vi "CoffeeMachine.vi"() -> ()   [LabVIEW 2020]
uses:
  Coffee Machine/ClusterConst.ctl
  Coffee Machine/Typedef/QueueOperations.ctl
  <vilib>/Utility/config.llb/Read Key (Double).vi
  <vilib>/Utility/config.llb/Read Key (I32).vi
  <vilib>/Utility/config.llb/Read Key (Boolean).vi
  <vilib>/Utility/config.llb/NI_LVConfig.lvlib
panel:
  out "error out":errorcluster
  in  "error in":errorcluster
  in  "Power":bool
  out "Total Cups":i32
  out "Elapsed Time":dbl
  out "Dispensing":bool
  out "Brewing":bool
  out "Grinding":bool
  out "Heating":bool
  out "Purging":bool
  out "Dispenser":dbl(slide) scale=0.0..10.0
  out "Chamber":dbl(slide) scale=0.0..10.0
  out "Low Milk":bool
  out "Low Bean":bool
  out "Low Water":bool
  out "Milk Level":dbl(slide) scale=0.0..100.0
  out "Bean Level":dbl(slide) scale=0.0..100.0
  out "Water Level":dbl(slide) scale=0.0..100.0
  in  "Type":i32(knob) scale=0.0..2.0
  in  "1-Carafe":bool
  in  "1- Cup":bool
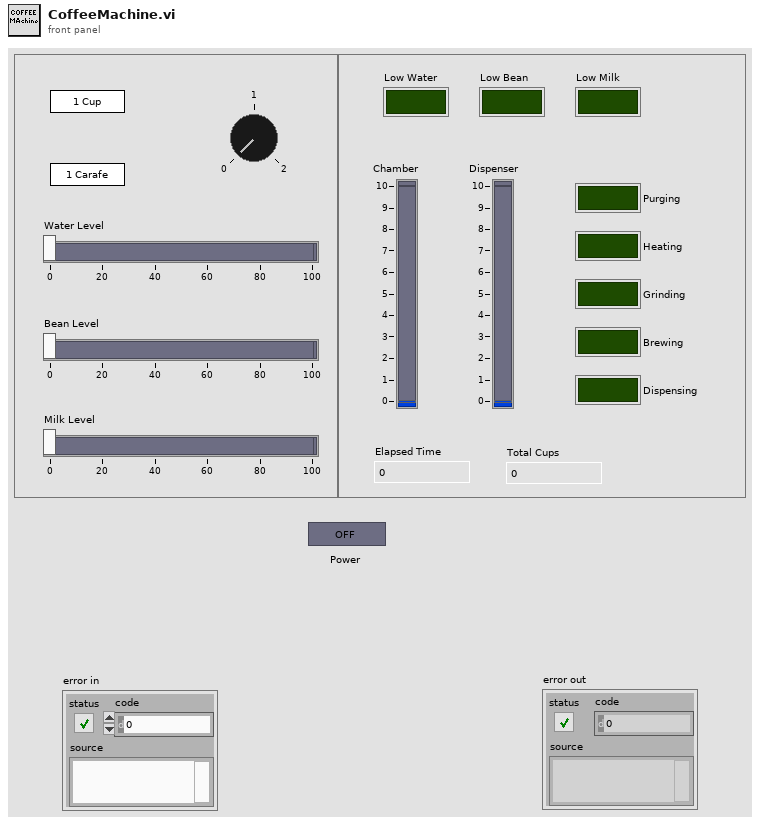
[diagram p1: front panel]
types:
  T1 = typedef "QueueOperations.ctl" = enum16{"Create", "Enqueue", "Enqueue N elements", "Dequeue", "Flush", "Release"}
  T2 = typedef "ClusterConst.ctl" = cluster{"1- Cup":bool, "1-Carafe":bool, "Water Level":dbl, "Bean Level":dbl, "Milk Level":dbl, "Purging":bool, "Heating":bool, "Grinding":bool, "Brewing":bool, "Dispensing":bool, "Chamber ":dbl, "Dispenser":dbl, "Low Water":bool, "Low Bean":bool, "Low Milk":bool, "Elapsed Time":dbl, "Total Cups":i32, "Power":bool, "Type":i32, "Level Array":dbl[], "Shutdown Status":bool, "Time Elapse":dbl, "Start Time":dbl, "Start 1 Seq":i32[], "Start 2 Seq":i32[], "Index":i32}
  T3 = typedef "NI_LVConfig.lvlib/Config Data RefNum.ctl" = refnum<k1>
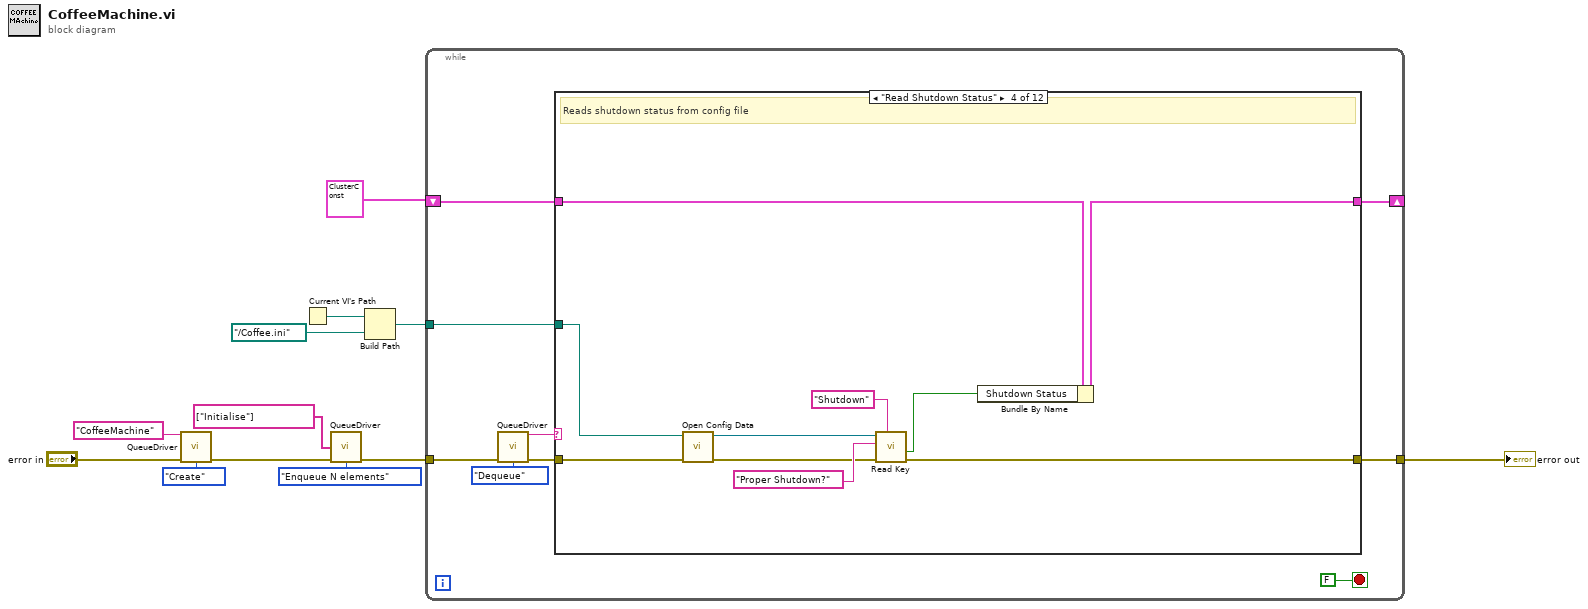
[diagram p0: block diagram]
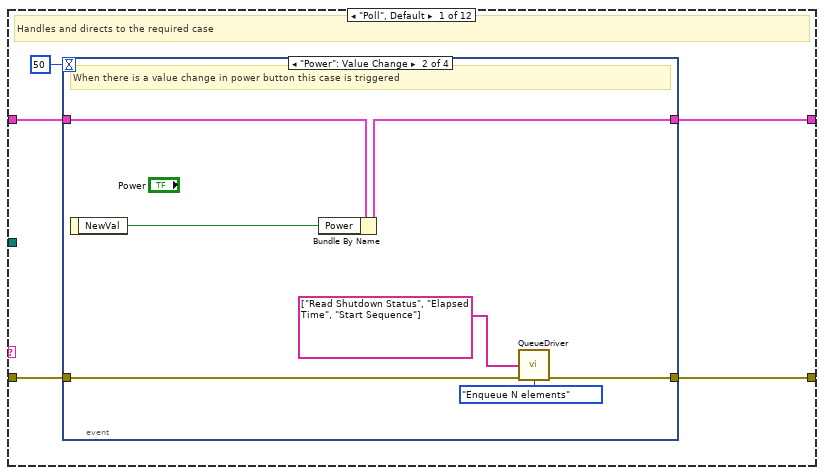
[diagram p2: hidden frame]
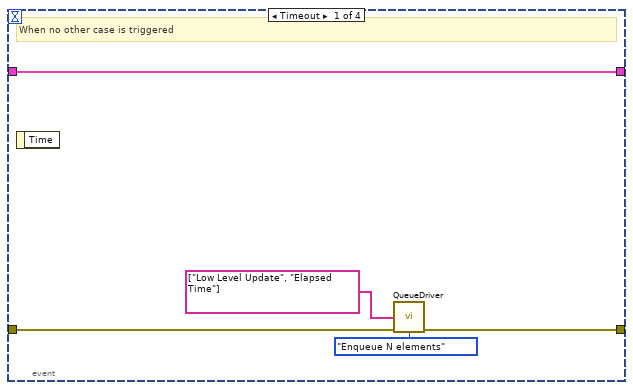
[diagram p3: hidden frame]
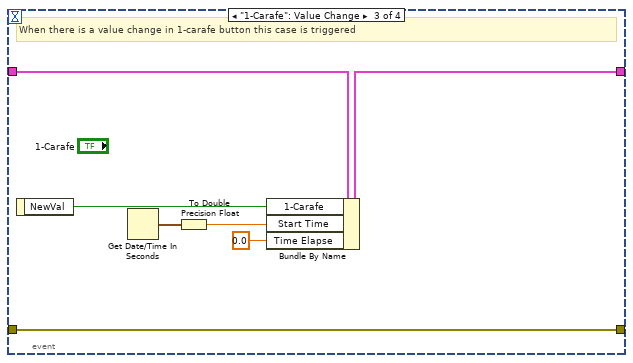
[diagram p4: hidden frame]
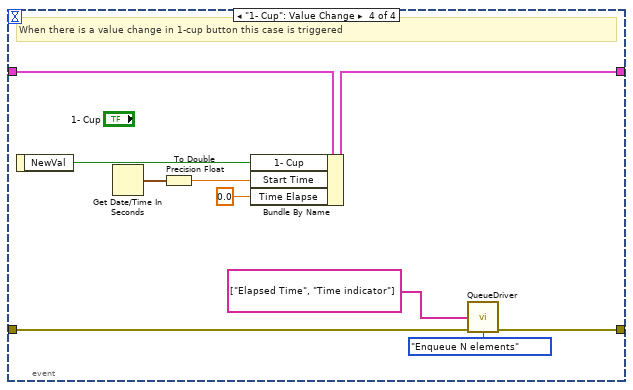
[diagram p5: hidden frame]
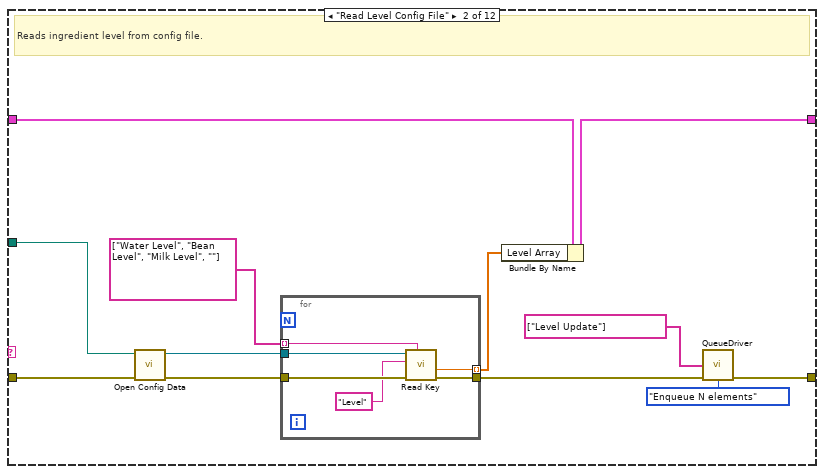
[diagram p6: hidden frame]
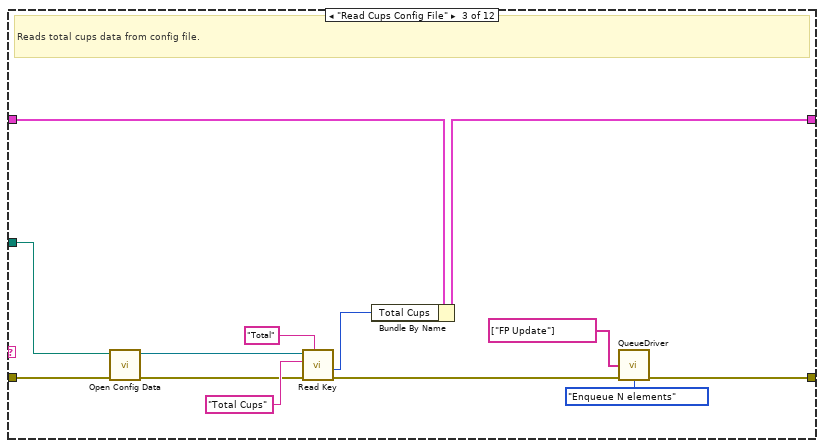
[diagram p7: hidden frame]
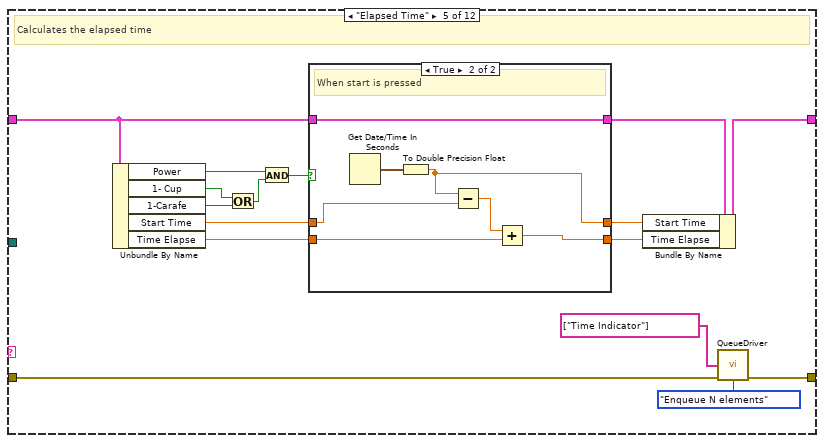
[diagram p8: hidden frame]
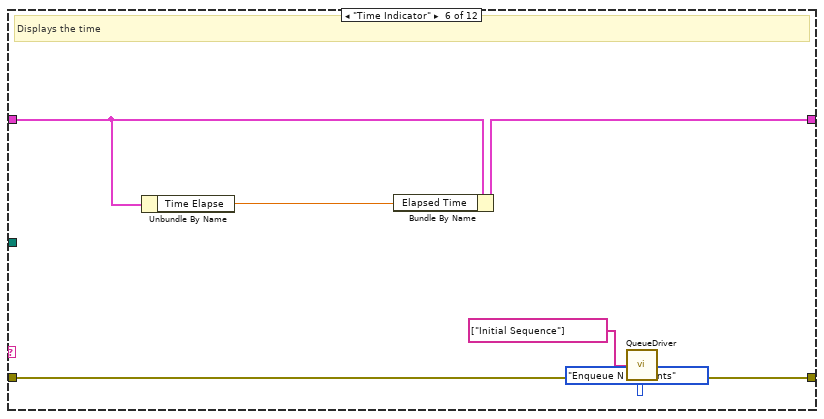
[diagram p10: hidden frame]
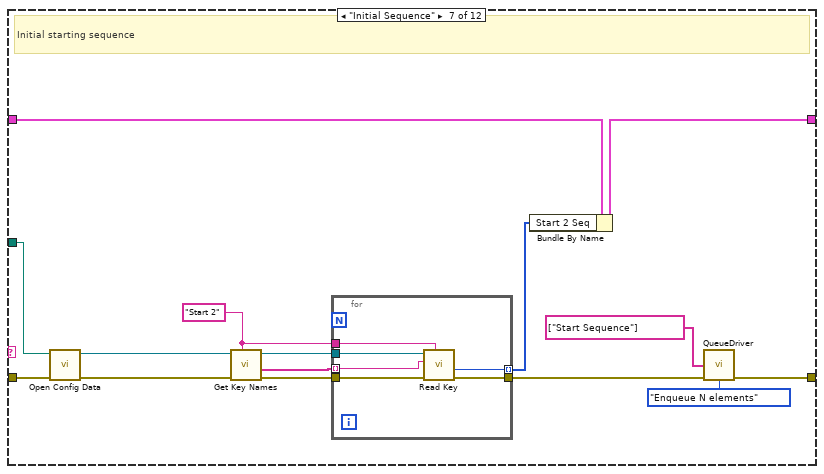
[diagram p11: hidden frame]
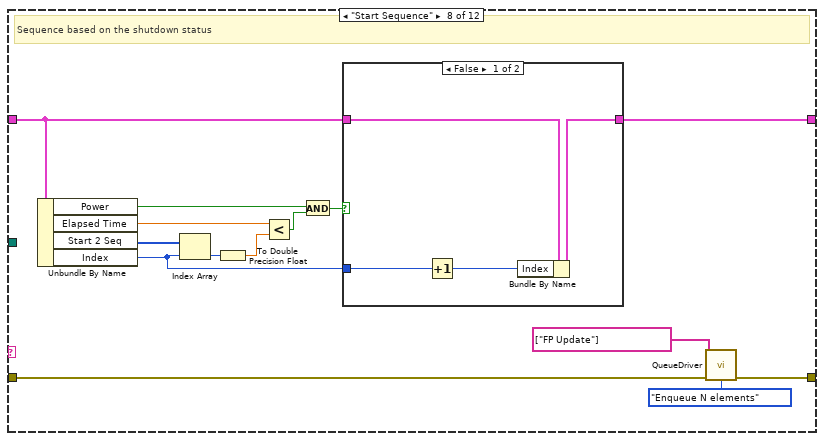
[diagram p12: hidden frame]
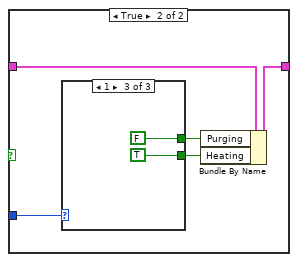
[diagram p13: hidden frame]
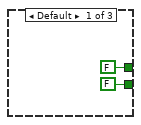
[diagram p14: hidden frame]
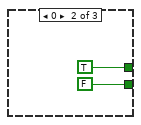
[diagram p15: hidden frame]
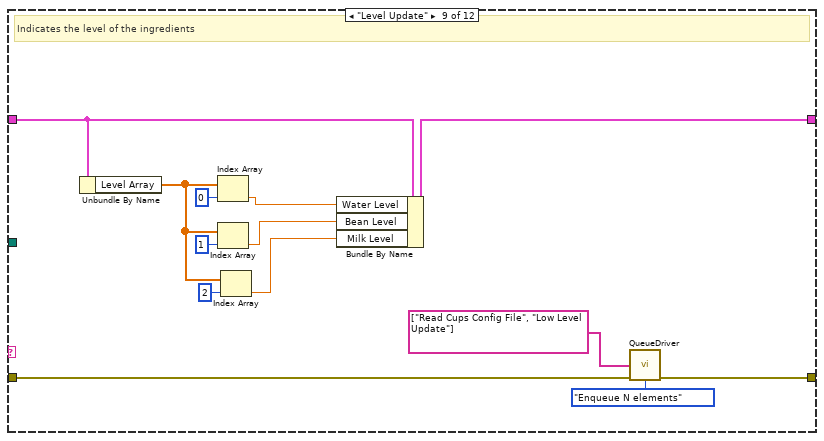
[diagram p16: hidden frame]
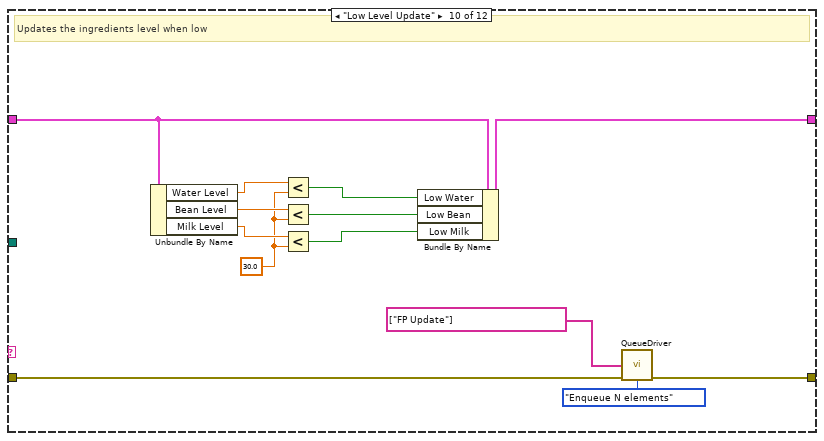
[diagram p17: hidden frame]
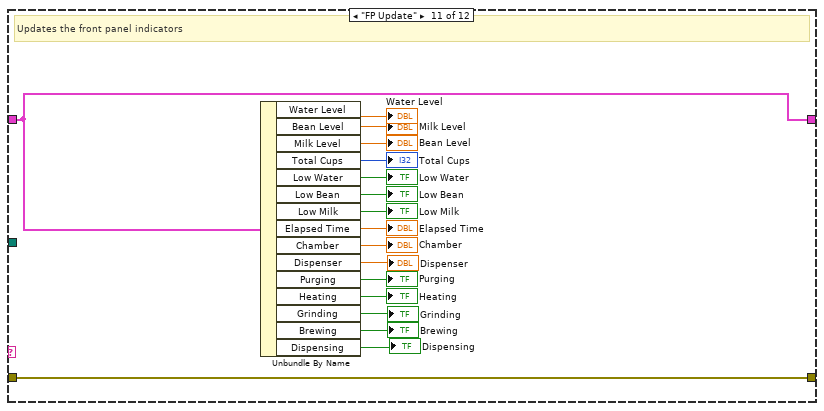
[diagram p18: hidden frame]
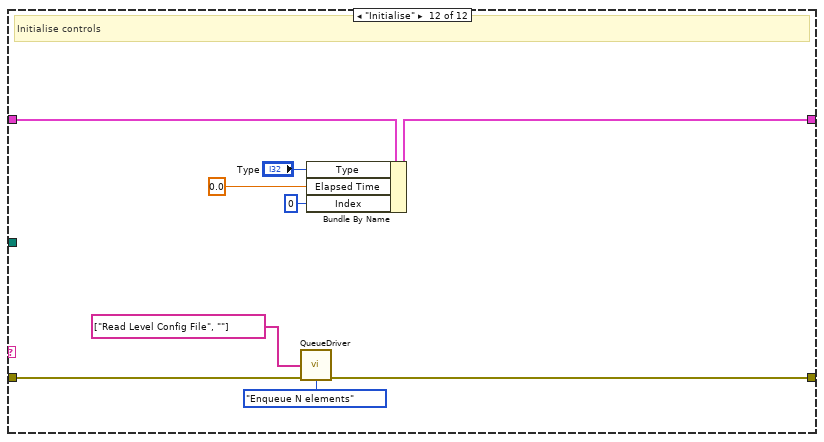
[diagram p19: hidden frame]
diagram:
  n1 = call "QueueDriver.vi"("Queue Name"="CoffeeMachine", "error in"="error in", "Queue Operations"=QueueOperations."Create") -> ("error out"=w8:errorcluster)  [unwired: 11 in, 1 out]
  n2 = Current VI's Path() -> (path=w4:path)
  n3 = call "QueueDriver.vi"("Array State"=string[] ["Initialise"], "error in"=w8, "Queue Operations"=QueueOperations."Enqueue N elements") -> ("error out"=w7:errorcluster)  [unwired: 11 in, 1 out]
  n4 = Build Path(base path=w4, name or relative path=path "../Coffee.ini") -> (appended path=w2:path)
  n5 = while {
    shift-right: [w16] -> _
    shift-left: T2 {"1- Cup"=TRUE, "1-Carafe"=FALSE, "Water Level"=0.0, "Bean Level"=0.0, "Milk Level"=0.0, "Purging"=FALSE, "Heating"=FALSE, "Grinding"=FALSE, "Brewing"=FALSE, "Dispensing"=FALSE, "Chamber "=0.0, "Dispenser"=0.0, "Low Water"=FALSE, "Low Bean"=FALSE, "Low Milk"=FALSE, "Elapsed Time"=0.0, "Total Cups"=0, "Power"=FALSE, "Type"=0, "Level Array"=[], "Shutdown Status"=FALSE, "Time Elapse"=0.0, "Start Time"=0.0, "Start 1 Seq"=[], "Start 2 Seq"=[], "Index"=0} -> [w17]
    tunnel: w7 -> [w21]
    tunnel: [w15] -> w1
    tunnel: w2 -> [w14]
    stop <- FALSE stop-if-true
    n6 = call "QueueDriver.vi"("error in"=w21, "Queue Operations"=QueueOperations."Dequeue") -> ("Dequeue State"=w18:string, "error out"=w20:errorcluster)  [unwired: 12 in]
    n7 = case shown="\"Read Shutdown Status\"" w18 {
      tunnel: w20 -> [w24 w65 w83 w91 w99 w124 w143 w155 w181 w194 w222 w227]
      tunnel: w17 -> [w26 w67 w86 w96 w110 w129 w144 w160 w192 w205 w221 w231]
      tunnel: [w25 w61 w79 w88 w108 w128 w135 w159 w187 w200 w221 w230] -> w16
      tunnel: [w23 w56 w75 w90 w98 w123 w130 w154 w180 w193 w222 w226] -> w15
      tunnel: w14 -> [_ w66 w81 w89 _ _ w142 _ _ _ _ _]
      frame "Poll", Default {
        # "Handles and directs to the required case"
        n8 = event shown="[1] \"Power\": Value Change" {
          selector: _ -> [_ _ _ _]
          dyn-events: _ -> [_ _ _ _]
          timeout: 50 -> [_ _ _ _]
          tunnel: w26 -> [w31 w38 w45 w55]
          tunnel: [w31 w37 w43 w54] -> w25
          tunnel: w24 -> [w28 w33 w44 w47]
          tunnel: [w27 w32 w44 w46] -> w23
          event Timeout {
            # "When no other case is triggered"
            n9 = event-data() -> ()  [unwired: 1 in, 1 out]
            n10 = call "QueueDriver.vi"("Array State"=string[] ["Low Level Update", "Elapsed Time"], "error in"=w28, "Queue Operations"=QueueOperations."Enqueue N elements") -> ("error out"=w27:errorcluster)  [unwired: 11 in, 1 out]
          }
          event "Power": Value Change {
            # "When there is a value change in power button this case is triggered"
            n11 = event-data() -> ("NewVal"=w36:bool)  [unwired: 1 in]
            n12 = Bundle By Name(cluster=w38, "Power"=w36) -> (w37:T2)
            n13 = call "QueueDriver.vi"("Array State"=string[] ["Read Shutdown Status", "Elapsed Time", "Start Sequence"], "error in"=w33, "Queue Operations"=QueueOperations."Enqueue N elements") -> ("error out"=w32:errorcluster)  [unwired: 11 in, 1 out]
          }
          event "1-Carafe": Value Change {
            # "When there is a value change in 1-carafe button this case is triggered"
            n14 = event-data() -> ("NewVal"=w42:bool)  [unwired: 1 in]
            n15 = Get Date/Time In Seconds() -> (seconds since 1Jan1904=w41:timestamp)
            n16 = To Double Precision Float(number=w41) -> (double precision float=w40:dbl)
            n17 = Bundle By Name(cluster=w45, "1-Carafe"=w42, "Start Time"=w40, "Time Elapse"=0.0 ("Elaspsed Time")) -> (w43:T2)
          }
          event "1- Cup": Value Change {
            # "When there is a value change in 1-cup button this case is triggered"
            n18 = event-data() -> ("NewVal"=w53:bool)  [unwired: 1 in]
            n19 = Get Date/Time In Seconds() -> (seconds since 1Jan1904=w52:timestamp)
            n20 = To Double Precision Float(number=w52) -> (double precision float=w51:dbl)
            n21 = Bundle By Name(cluster=w55, "1- Cup"=w53, "Start Time"=w51, "Time Elapse"=0.0 ("Elaspsed Time")) -> (w54:T2)
            n22 = call "QueueDriver.vi"("Array State"=string[] ["Elapsed Time", "Time indicator"], "error in"=w47, "Queue Operations"=QueueOperations."Enqueue N elements") -> ("error out"=w46:errorcluster)  [unwired: 11 in, 1 out]
          }
        }
      }
      frame "Read Level Config File" {
        # "Reads ingredient level from config file."
        n23 = call <vilib>:"Open Config Data.vi"("error in (no error)"=w65, "configuration file path"=w66) -> ("error out"=w64:errorcluster, "refnum"=w63:T3)  [unwired: 7 in, 1 out]
        n24 = for {
          tunnel: w64 -> [w72]
          tunnel: [w73] -> w57
          tunnel: w63 -> [w71]
          tunnel: string[] ["Water Level", "Bean Level", "Milk Level", ""] ("section") -> [w70] mode=indexing
          tunnel: [w69] -> w60 mode=indexing
          n25 = call-poly <vilib>:"Read Key.vi"("section"=w70, "error in (no error)"=w72, "key"="Level", "refnum"=w71) -> ("error out"=w73:errorcluster, "value"=w69:dbl)  [unwired: 4 in, 2 out]
        }
        n26 = Bundle By Name(cluster=w67, "Level Array"=w60) -> (w61:T2)
        n27 = call "QueueDriver.vi"("Array State"=string[] ["Level Update"], "error in"=w57, "Queue Operations"=QueueOperations."Enqueue N elements") -> ("error out"=w56:errorcluster)  [unwired: 11 in, 1 out]
      }
      frame "Read Cups Config File" {
        # "Reads total cups data from config file."
        n28 = call <vilib>:"Open Config Data.vi"("error in (no error)"=w83, "configuration file path"=w81) -> ("error out"=w82:errorcluster, "refnum"=w80:T3)  [unwired: 7 in, 1 out]
        n29 = call-poly <vilib>:"Read Key.vi"("section"="Total", "error in (no error)"=w82, "key"="Total Cups", "refnum"=w80) -> ("error out"=w76:errorcluster, "value"=w78:i32)  [unwired: 4 in, 2 out]
        n30 = Bundle By Name(cluster=w86, "Total Cups"=w78) -> (w79:T2)
        n31 = call "QueueDriver.vi"("Array State"=string[] ["FP Update"], "error in"=w76, "Queue Operations"=QueueOperations."Enqueue N elements") -> ("error out"=w75:errorcluster)  [unwired: 11 in, 1 out]
      }
      frame "Read Shutdown Status" {
        # "Reads shutdown status from config file"
        n32 = call <vilib>:"Open Config Data.vi"("error in (no error)"=w91, "configuration file path"=w89) -> ("error out"=w93:errorcluster, "refnum"=w92:T3)  [unwired: 7 in, 1 out]
        n33 = call-poly <vilib>:"Read Key.vi"("section"="Shutdown", "error in (no error)"=w93, "key"="Proper Shutdown?", "refnum"=w92) -> ("error out"=w90:errorcluster, "value"=w87:bool)  [unwired: 4 in, 2 out]
        n34 = Bundle By Name(cluster=w96, "Shutdown Status"=w87) -> (w88:T2)
      }
      frame "Elapsed Time" {
        # "Calculates the elapsed time"
        n35 = Unbundle By Name(w110) -> ("Power"=w102:bool, "1- Cup"=w112:bool, "1-Carafe"=w111:bool, "Start Time"=w107:dbl, "Time Elapse"=w106:dbl)
        n36 = Or(x=w112, y=w111) -> (x .or. y?=w103:bool)
        n37 = And(x=w102, y=w103) -> (x .and. y?=w101:bool)
        n38 = case shown="True" w101 {
          tunnel: w110 -> [w115 w122]
          tunnel: [w115 w122] -> w109
          tunnel: w107 -> [w114 w120]
          tunnel: w106 -> [w113 w119]
          tunnel: [w114 w116] -> w105
          tunnel: [w113 w118] -> w104
          frame False {
            # "When start not pressed"
          }
          frame True {
            # "When start is pressed"
            n39 = Get Date/Time In Seconds() -> (seconds since 1Jan1904=w121:timestamp)
            n40 = To Double Precision Float(number=w121) -> (double precision float=w116:dbl)
            n41 = Subtract(x=w116, y=w120) -> (x-y=w117:dbl)
            n42 = Add(x=w117, y=w119) -> (x+y=w118:dbl)
          }
        }
        n43 = Bundle By Name(cluster=w109, "Start Time"=w105, "Time Elapse"=w104) -> (w108:T2)
        n44 = call "QueueDriver.vi"("Array State"=string[] ["Time Indicator"], "error in"=w99, "Queue Operations"=QueueOperations."Enqueue N elements") -> ("error out"=w98:errorcluster)  [unwired: 11 in, 1 out]
      }
      frame "Time Indicator" {
        # "Displays the time"
        n45 = Unbundle By Name(w129) -> ("Time Elapse"=w127:dbl)
        n46 = Bundle By Name(cluster=w129, "Elapsed Time"=w127) -> (w128:T2)
        n47 = call "QueueDriver.vi"("Array State"=string[] ["Initial Sequence"], "error in"=w124, "Queue Operations"=QueueOperations."Enqueue N elements") -> ("error out"=w123:errorcluster)  [unwired: 11 in, 1 out]
      }
      frame "Initial Sequence" {
        w136 = "Start 2" ("section")
        # "Initial starting sequence"
        n48 = call <vilib>:"Open Config Data.vi"("error in (no error)"=w143, "configuration file path"=w142) -> ("error out"=w141:errorcluster, "refnum"=w140:T3)  [unwired: 7 in, 1 out]
        n49 = call <vilib>:"Get Key Names.vi"("section"=w136, "error in (no error)"=w141, "refnum"=w140) -> ("error out"=w139:errorcluster, "key names"=w137:string[], "refnum out"=w138:T3)  [unwired: 5 in, 1 out]
        n50 = for {
          tunnel: w139 -> [w149]
          tunnel: [w150] -> w131
          tunnel: w138 -> [w148]
          tunnel: [w147] -> w134 mode=indexing
          tunnel: w137 -> [w146] mode=indexing
          tunnel: w136 -> [w145]
          n51 = call-poly <vilib>:"Read Key.vi"("section"=w145, "error in (no error)"=w149, "key"=w146, "refnum"=w148) -> ("error out"=w150:errorcluster, "value"=w147:i32)  [unwired: 4 in, 2 out]
        }
        n52 = Bundle By Name(cluster=w144, "Start 2 Seq"=w134) -> (w135:T2)
        n53 = call "QueueDriver.vi"("Array State"=string[] ["Start Sequence"], "error in"=w131, "Queue Operations"=QueueOperations."Enqueue N elements") -> ("error out"=w130:errorcluster)  [unwired: 11 in, 1 out]
      }
      frame "Start Sequence" {
        # "Sequence based on the shutdown status"
        n54 = Unbundle By Name(w160) -> ("Power"=w152:bool, "Elapsed Time"=w163:dbl, "Start 2 Seq"=w164:i32[], "Index"=w158:i32)
        n55 = Index Array(array=w164, index=w158) -> (element=w162:i32)
        n56 = To Double Precision Float(number=w162) -> (double precision float=w161:dbl)
        n57 = Less?(x=w163, y=w161) -> (x < y?=w153:bool)
        n58 = And(x=w152, y=w153) -> (x .and. y?=w151:bool)
        n59 = case shown="False" w151 {
          tunnel: w160 -> [w168 w173]
          tunnel: [w167 w172] -> w159
          tunnel: w158 -> [w166 w169]
          frame False {
            n60 = Increment(x=w166) -> (x+1=w165:i32)
            n61 = Bundle By Name(cluster=w168, "Index"=w165) -> (w167:T2)
          }
          frame True {
            n62 = case shown="1" w169 {
              tunnel: [FALSE ("Purging") TRUE ("Purging") FALSE ("Purging")] -> w171
              tunnel: [FALSE ("Heating") FALSE ("Heating") TRUE ("Heating")] -> w170
              frame Default {
              }
              frame 0 {
              }
              frame 1 {
              }
            }
            n63 = Bundle By Name(cluster=w173, "Purging"=w171, "Heating"=w170) -> (w172:T2)
          }
        }
        n64 = call "QueueDriver.vi"("Array State"=string[] ["FP Update"], "error in"=w155, "Queue Operations"=QueueOperations."Enqueue N elements") -> ("error out"=w154:errorcluster)  [unwired: 11 in, 1 out]
      }
      frame "Level Update" {
        # "Indicates the level of the ingredients"
        n65 = Unbundle By Name(w192) -> ("Level Array"=w191:dbl[])
        n66 = Index Array(array=w191, index=0) -> (element=w186:dbl)
        n67 = Index Array(array=w191, index=1) -> (element=w185:dbl)
        n68 = Index Array(array=w191, index=2) -> (element=w184:dbl)
        n69 = Bundle By Name(cluster=w192, "Water Level"=w186, "Bean Level"=w185, "Milk Level"=w184) -> (w187:T2)
        n70 = call "QueueDriver.vi"("Array State"=string[] ["Read Cups Config File", "Low Level Update"], "error in"=w181, "Queue Operations"=QueueOperations."Enqueue N elements") -> ("error out"=w180:errorcluster)  [unwired: 11 in, 1 out]
      }
      frame "Low Level Update" {
        w201 = 30.0 ("y")
        # "Updates the ingredients level when low"
        n71 = Unbundle By Name(w205) -> ("Water Level"=w204:dbl, "Bean Level"=w203:dbl, "Milk Level"=w202:dbl)
        n72 = Less?(x=w204, y=w201) -> (x < y?=w199:bool)
        n73 = Less?(x=w203, y=w201) -> (x < y?=w198:bool)
        n74 = Less?(x=w202, y=w201) -> (x < y?=w197:bool)
        n75 = Bundle By Name(cluster=w205, "Low Water"=w199, "Low Bean"=w198, "Low Milk"=w197) -> (w200:T2)
        n76 = call "QueueDriver.vi"("Array State"=string[] ["FP Update"], "error in"=w194, "Queue Operations"=QueueOperations."Enqueue N elements") -> ("error out"=w193:errorcluster)  [unwired: 11 in, 1 out]
      }
      frame "FP Update" {
        # "Updates the front panel indicators"
        n77 = Unbundle By Name(w221) -> ("Water Level"=→"Water Level":dbl, "Bean Level"=→"Milk Level":dbl, "Milk Level"=→"Bean Level":dbl, "Total Cups"=→"Total Cups":i32, "Low Water"=→"Low Water":bool, "Low Bean"=→"Low Bean":bool, "Low Milk"=→"Low Milk":bool, "Elapsed Time"=→"Elapsed Time":dbl, "Chamber"=→"Chamber":dbl, "Dispenser"=→"Dispenser":dbl, "Purging"=→"Purging":bool, "Heating"=→"Heating":bool, "Grinding"=→"Grinding":bool, "Brewing"=→"Brewing":bool, "Dispensing"=→"Dispensing":bool)
      }
      frame "Initialise" {
        # "Initialise controls"
        n78 = call "QueueDriver.vi"("Array State"=string[] ["Read Level Config File", ""], "error in"=w227, "Queue Operations"=QueueOperations."Enqueue N elements") -> ("error out"=w226:errorcluster)  [unwired: 11 in, 1 out]
        n79 = Bundle By Name(cluster=w231, "Type"="Type", "Elapsed Time"=0.0, "Index"=0) -> (w230:T2)
      }
    }
  }
  "error out" <- w1
